vi "Get Selected Cell Location.vi"(9 "column":i32, 10 "row":i32, 11 "DataGridView in":refnum<class "DataGridView.lvclass">) -> (2 "Coords":T1, 3 "DataGridView out":refnum<class "DataGridView.lvclass">)   [LabVIEW 2013, in "DataGrid.lvlib" / "DataGridView.lvclass"]
uses:
  DataGridView.lvclass
  <vilib>/Utility/miscctls.llb/LVPoint32TypeDef.ctl
  DataGridView.lvclass/DataGridView.ctl
  System.Windows.Forms
  System.Drawing
  Properties/Read DataGridView.vi
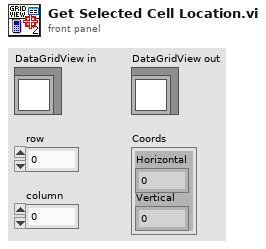
[diagram p1: front panel]
types:
  T1 = typedef "LVPoint32TypeDef.ctl" = cluster{"Horizontal":i32, "Vertical":i32}
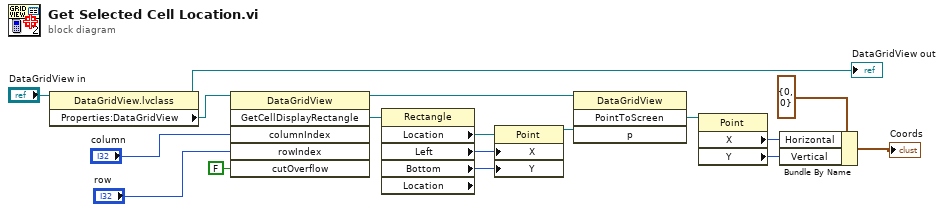
[diagram p0: block diagram]
diagram:
  n1 = property class="DataGridView.lvclass"(reference="DataGridView in") -> (reference out=→"DataGridView out":refnum<class "DataGridView.lvclass">, "Properties:DataGridView"=w6:refnum<k24>)  [unwired: 1 in, 1 out]
  n2 = invoke class="DataGridView" method="GetCellDisplayRectangle"(reference=w6, "columnIndex"="column", "rowIndex"="row", "cutOverflow"=FALSE) -> (reference out=w16:refnum<k24>, "GetCellDisplayRectangle"=w2:refnum<k24>)  [unwired: 2 in, 4 out]
  n3 = property class="Rectangle" props=["Location", "Left", "Bottom", "Location"](reference=w2) -> ("Location"=w15:refnum<k24>, "Left"=w14:i32, "Bottom"=w9:i32)  [unwired: 1 in, 3 out]
  n4 = property class="Point"(reference=w15, "X"=w14, "Y"=w9) -> (reference out=w8:refnum<k24>)  [unwired: 1 in, 1 out]
  n5 = invoke class="DataGridView" method="PointToScreen"(reference=w16, "p"=w8) -> ("PointToScreen"=w7:refnum<k24>)  [unwired: 2 in, 3 out]
  n6 = property class="Point"(reference=w7) -> ("X"=w11:i32, "Y"=w12:i32)  [unwired: 1 in, 2 out]
  n7 = Bundle By Name(cluster=T1 {"Horizontal"=0, "Vertical"=0} ("Coords"), "Horizontal"=w11, "Vertical"=w12) -> (→"Coords":T1)
